vi "move to cache.vi"(7 "Time Stamp":timestamp, 8 "sample counter":i32, 10 "data table in":T1, 11 "cache in":T2) -> (2 "data table out":T1, 3 "cache out":T2)   [LabVIEW 2013, in "Binary datalogger runtime.lvclass"]
uses:
  Binary datalogger runtime.lvclass
  data cache.ctl
  <vilib>/NI/Tag Bus/table/data table.ctl
  <vilib>/NI/Tag Bus/table/data table.lvlib
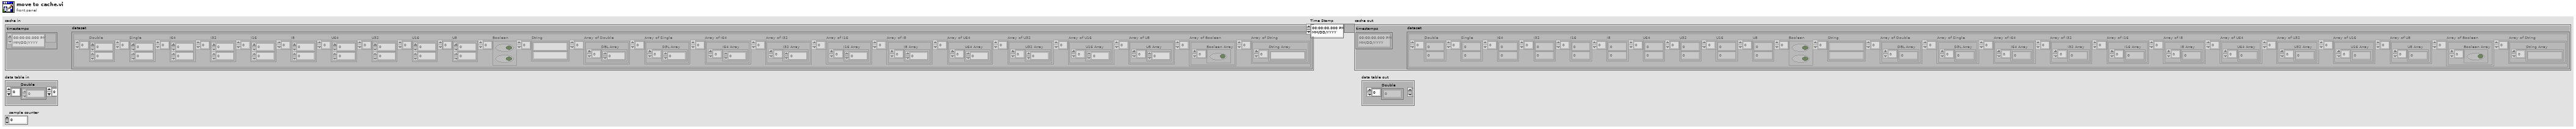
[diagram p1: front panel]
types:
  T1 = typedef "tag bus.lvlib/data table.lvlib/data table.ctl" = cluster{"Double":dbl[], "Single":sgl[], "I64":i64[], "I32":i32[], "I16":i16[], "I8":i8[], "U64":u64[], "U32":u32[], "U16":u16[], "U8":u8[], "Boolean":bool[], "String":string[], "Array of Double":cluster{"DBL Array":dbl[]}[], "Array of Single":cluster{"SGL Array":sgl[]}[], "Array of I64":cluster{"I64 Array":i64[]}[], "Array of I32":cluster{"I32 Array":i32[]}[], "Array of I16":cluster{"I16 Array":i16[]}[], "Array of I8":cluster{"I8 Array":i8[]}[], "Array of U64":cluster{"U64 Array":u64[]}[], "Array of U32":cluster{"U32 Array":u32[]}[], "Array of U16":cluster{"U16 Array":u16[]}[], "Array of U8":cluster{"U8 Array":u8[]}[], "Array of Boolean":cluster{"Boolean Array":bool[]}[], "Array of String":cluster{"String Array":string[]}[]}
  T2 = typedef "Binary datalogger runtime.lvclass/data cache.ctl" = cluster{"timestamps":timestamp[], "dataset":T1[]}
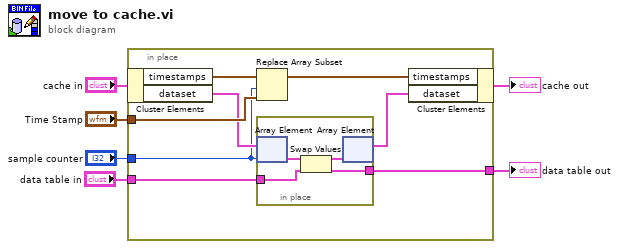
[diagram p0: block diagram]
diagram:
  n1 = in-place {
    in-place-border: "sample counter" -> [w10]
    in-place-border: "Time Stamp" -> [w12]
    in-place-border: "data table in" -> [w8]
    in-place-border: [w7] -> w1
    n2 = in-place-cluster #1("cache in") -> ("timestamps"=w14:timestamp[], "dataset"=w11:T1[])
    n3 = Replace Array Subset(array=w14, new element=w12, index=w10) -> (w13:timestamp[])
    n4 = in-place {
      in-place-border: w8 -> [w16]
      in-place-border: [w15] -> w7
      n5 = in-place-array #2(w11, w10) -> (w18:T1)
      n6 = Swap Values(12:w18, 14:w16) -> (1:w17:T1, 3:w15:T1)  [unwired: 1 in]
      n7 = in-place-array #2(w17) -> (w9:T1[])  [unwired: 1 out]
    }
    n8 = in-place-cluster #1("timestamps"=w13, "dataset"=w9) -> (→"cache out":T2)
  }
  "data table out" <- w1
